vi "Close.vi"(8 "error in (no error)":errorcluster, 11 "Comdel in":refnum<class "PL Lotis TII LS.lvclass">) -> (0 "error out":errorcluster)   [LabVIEW 2015, in "PL Lotis TII LS.lvclass"]
doc: "Closes connection to device."
uses:
  PL Lotis TII LS.lvclass
  PL Lotis TII LS.lvclass/PL Lotis TII LS.ctl
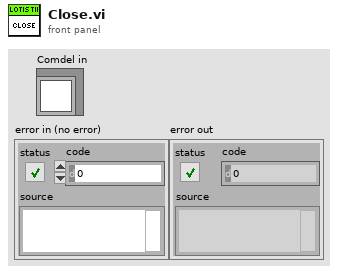
[diagram p1: front panel]
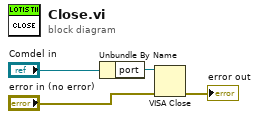
[diagram p0: block diagram]
diagram:
  n1 = Unbundle By Name("Comdel in") -> ("port"=w3:refnum<visa-resource-name>)
  n2 = VISA Close(VISA resource name=w3, error in (no error)="error in (no error)") -> (error out=→"error out":errorcluster)
